vi "Save Server Configuration.vi"(8 "error in (no error)":errorcluster) -> (0 "error out":errorcluster)   [LabVIEW 2024]
doc: "Saves server configurations to the configuration file."
uses:
  Globals/Global - Server.vi
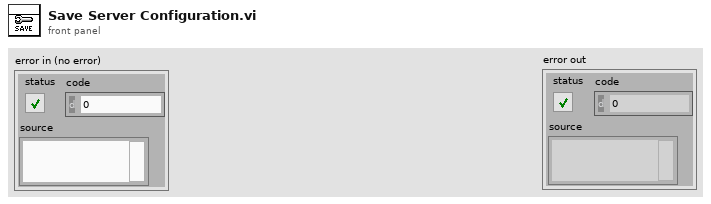
[diagram p1: front panel]
types:
  T1 = typedef "System Configuration.ctl" = cluster{"Name":string, "Description":string, "Logging Computer Name":string, "Logging Database Name":string, "Logging Database Path":path, "Archive Computer Name":string, "Archive Database Name":string, "Archive Database Path":path, "Lifespan (days)":u32, "Archive Enabled":bool, "Archive Interval (hours)":u32, "Subsystems":T2[]}
  T2 = typedef "Subsystem Configuration.ctl" = cluster{"Name":string, "Root URL":refnum<k21>}
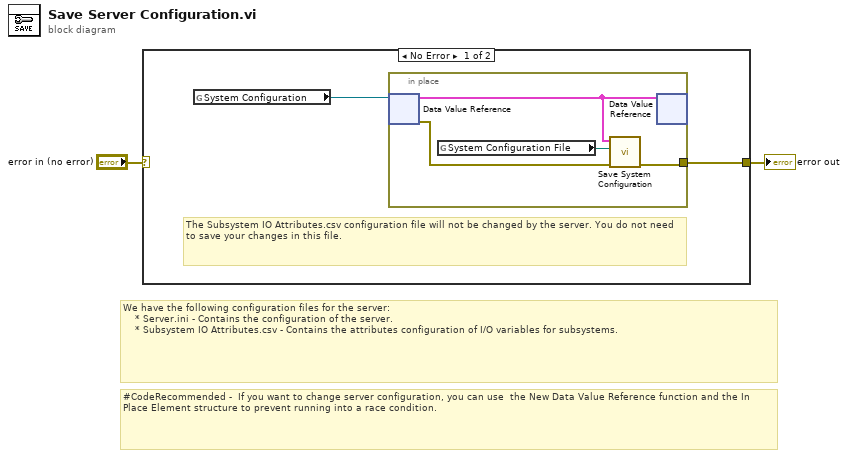
[diagram p0: block diagram]
diagram:
  # "#CodeRecommended -  If you want to change server configuration, you can use  the New Data Value Reference function and the In Place Element structure to prevent running into a race condition."
  # "We have the following configuration files for the server:\n    * Server.ini - Contains the configuration of the server.\n    * Subsystem IO Attributes.csv - Contains the attributes configuration of I/O variables for subsystems."
  n1 = case shown="No Error" "error in (no error)" {
    selector: "error in (no error)" -> [_ w9]
    tunnel: [w3 w9] -> w1
    frame No Error {
      # "The Subsystem IO Attributes.csv configuration file will not be changed by the server. You do not need to save your changes in this file."
      n2 = global read "Global - Server.vi" "System Configuration"() -> (w4:refnum<data-value>)
      n3 = in-place {
        in-place-border: [w8] -> w3
        n4 = in-place-dvr #1(w4) -> (w6:T1, w5:errorcluster)
        n5 = global read "Global - Server.vi" "System Configuration File"() -> (w7:path)
        n6 = call "Save System Configuration.vi"("error in (no error)"=w5, "System Configuration File Path"=w7, "System Configuration"=w6) -> ("error out"=w8:errorcluster)  [unwired: 8 in]
        n7 = in-place-dvr #1(w6) -> ()  [unwired: 2 out]
      }
    }
    frame Error {
    }
  }
  "error out" <- w1
